vi "Regler FT-IR.vi"(7 "Index":i32, 8 "Fehler":errorcluster caption="Fehler (Eingang)") -> (0 "Fehler (Ausgang)":errorcluster)   [LabVIEW 2020, in "Regler.lvlib" / "Druckregler.lvlib"]
uses:
  Druckregler.lvlib
  Verwaltung/Verwaltung - cRIO.lvlib
  Aktionen Param. Druckregler.ctl
  Visualisierungs Elemente/Zahlen-Eingabefeld.ctl
  Allgemein/Allgemein.lvlib
  Allgemein/Aktionen FGV Dichtheitstest.ctl
  Aktionen Interne Werte.ctl
  Konfig-Dateien/Konfig-Dateien.lvlib
  Verwaltung/FGV IN Aktionen.ctl
  Konfig-Dateien/FGV Betriebsdaten Aktionen.ctl
  Verwaltung/FGV OUT Aktionen.ctl
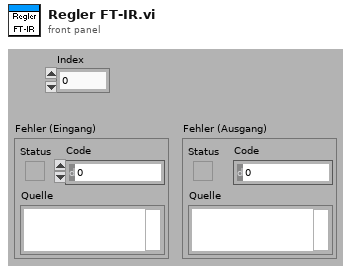
[diagram p1: front panel]
types:
  T1 = typedef "Verwaltung - cRIO.lvlib/FGV OUT Aktionen.ctl" = enum16{"lesen", "ANA OUT", "DO 0-31", "DO 32-47"}
  T2 = typedef "Konfig-Dateien.lvlib/FGV Betriebsdaten Aktionen.ctl" = enum16{"lesen", "Anlagengrenzw.", "PID Param.", "Sonstige", "Sensor Para."}
  T3 = typedef "Verwaltung - cRIO.lvlib/FGV IN Aktionen.ctl" = enum16{"lesen", "DI", "AI", "Fühler Br.", "TC", "Fühler Br. TC"}
  T4 = typedef "Regler.lvlib/Druckregler.lvlib/Aktionen Interne Werte.ctl" = enum16{"lesen", "FT-IR", "Ausgang", "Pumpe", "laden", "speichern", "Änderung?", "Druck Kalter Block", "Dichtheitstest"}
  T5 = typedef "Allgemein.lvlib/Aktionen FGV Dichtheitstest.ctl" = enum16{"lesen", "schreiben"}
  T6 = typedef "Zahlen-Eingabefeld.ctl" = sgl
  T7 = typedef "Regler.lvlib/Druckregler.lvlib/Aktionen Param. Druckregler.ctl" = enum16{"lesen", "schreiben", "Regler FT-IR", "Regler Ausgang", "Regler Durchfluss", "Regler PMA", "Regler NDIR", "Regler Filterblock", "Regler Gaskühler", "Regler Kalter Block"}
  T8 = typedef "Anlagengrenzwerte.lvlib/Anlagen-Grenzwerte Anzeige.ctl" = cluster{"Eingangsdruck FT-IR:":T9, "Durchfluss FT-IR:":T9, "Druck Ausgang:":T9, "Druck Kalter Block:":T9, "Heizleitungen intern:":T9, "Heizleitung zu FT-IR:":T9, "Heizung Filterblock:":T9, "Heizung Pumpe:":T9, "Heizleitung Extern SP1:":T9, "Heizleitung Extern SP2:":T9, "FT-IR Heizung Messzelle:":T9, "Schaltschranktemperatur:":T9, "Gaskühler:":T9, "Heizung VFE 2:":T9}
  T9 = typedef "Anlagengrenzwerte.lvlib/Anlagen-Parameter Anzeige.ctl" = cluster{"Sollwert":sgl, "Warn-Min":sgl, "Warn-Max":sgl, "Abschalt-Min":sgl, "Abschalt-Max":sgl, "Regler":u16}
  T10 = cluster{"AI0: Durchfluss FT-IR":sgl, "AI1: Druck Ausgang":sgl, "AI2: Umgebungsdruck":sgl, "AI3: Druck FT-IR":sgl, "AI4: Druck CalGas":sgl, "AI5: Reserve":sgl, "AI6: Reserve":sgl, "AI7: Reserve":sgl, "Rohwert Durchfluss FT-IR":sgl, "Rohwert Druck Ausgang":sgl, "Rohwert Umgebungsdruck":sgl, "Rohwert Druck FT-IR":sgl, "Schaltschrank":sgl, "Filter":sgl, "Pumpe":sgl, "HL BMP zu Filter":sgl, "HL zu FT-IR":sgl, "HL Extern SP1":sgl, "Reserve":sgl, "Reserve":sgl, "Reserve":sgl, "Reserve":sgl, "Reserve":sgl, "Reserve":sgl, "FT-IR":sgl, "Reserve":sgl, "Reserve":sgl, "Reserve":sgl}
  T11 = typedef "Verwaltung - cRIO.lvlib/Digital Ausgaenge 0-31.ctl" = cluster{"O0: Druckluft Versorgung":bool, "O1: (FB Eingang 1)":bool, "O2: Kühlung FT-IR EIN":bool, "O3: (FB Bypass)":bool, "O4: (FB CalGas)":bool, "O5: (FB spülen/UL)":bool, "O6: (FB zum FT-IR)":bool, "O7: (FB zum FID)":bool, "O8: (FB Reserve)":bool, "O9: (FB Reserve)":bool, "O10: (FB Umgebungsluft FID)":bool, "O11: (FB zum Gaskühler)":bool, "O12: FB Stickstoff zu FT-IR":bool, "O13: (FB Druckluft/UL)":bool, "O14: (Purifier deaktivieren)":bool, "O15: (Umschaltung Purifier/Stickstoff)":bool, "O16: N2 Einblasung":bool, "O17: LSP LN2 Nachfüllung":bool, "O18: (Reserve)":bool, "O19: (Pumpe Eingang1)":bool, "O20: (Pumpe Eingang2)":bool, "O21: (Pumpe Spülen1)":bool, "O22: (Pumpe Spülen2)":bool, "O23: (Reserve)":bool, "O24: CalGas 1":bool, "O25: CalGas 2":bool, "O26: CalGas 3":bool, "O27: Stickstoff aufschalten":bool, "O28: CG zu PNS":bool, "O29: FTIR Standby Spülung":bool, "O30: (Reserve)":bool, "O31: (Purifier regenerieren)":bool}
  T12 = cluster{"Numerisch":sgl, "Numerisch":sgl, "Numerisch":sgl, "Numerisch":sgl, "Numerisch":sgl}
  T13 = typedef "Regler.lvlib/Druckregler.lvlib/Regler Interne Werte.ctl" = cluster{"PV":sgl, "D-action":sgl, "Error":sgl, "I-action":sgl, "OUT":sgl}
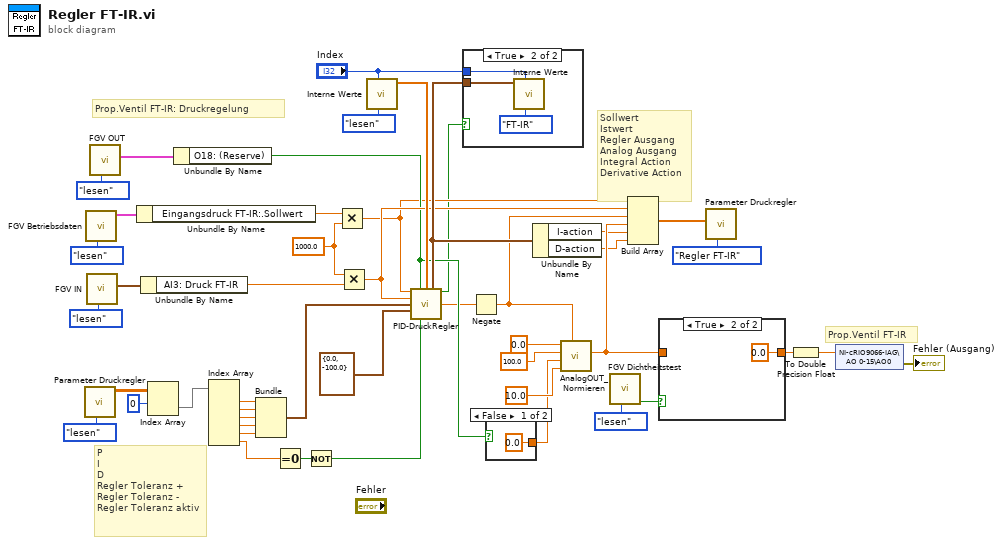
[diagram p0: block diagram]
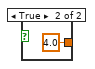
[diagram p4: hidden frame]
diagram:
  w25 = T6 1000.0 ("y")
  # "Prop.Ventil FT-IR"
  # "Prop.Ventil FT-IR: Druckregelung"
  # "Sollwert\nIstwert\nRegler Ausgang\nAnalog Ausgang\nIntegral Action\nDerivative Action"
  # "P\nI\nD\nRegler Toleranz +\nRegler Toleranz -\nRegler Toleranz aktiv"
  n1 = call "Parameter Druckregler.vi"("Aktionen"=Aktionen_Param._Druckregler."lesen") -> ("Regleparameter"=w30:sgl[][])  [unwired: 7 in, 3 out]
  n2 = call "FGV Betriebsdaten.vi"("Aktionen"=FGV_Betriebsdaten_Aktionen."lesen") -> ("Anlagen-Grenzwerte"=w2:T8)  [unwired: 7 in, 3 out]
  n3 = call "FGV IN.vi"("Aktion"=FGV_IN_Aktionen."lesen") -> ("Analog Eingänge"=w1:T10)  [unwired: 8 in, 2 out]
  n4 = call "FGV OUT.vi"("Aktion"=FGV_OUT_Aktionen."lesen") -> ("DO 0-31"=w3:T11)  [unwired: 7 in, 3 out]
  n5 = Unbundle By Name(w2) -> ("Eingangsdruck FT-IR:.Sollwert"=w26:sgl)
  n6 = Unbundle By Name(w1) -> ("AI3: Druck FT-IR"=w24:sgl)
  n7 = Index Array(array=w30, index (row)=0 ("Deaktivierter Index (Spalte)")) -> (element=w29:sgl[])  [unwired: 1 in]
  n8 = Unbundle By Name(w3) -> ("O18: (Reserve)"=w16:bool)
  n9 = Index Array(array=w29) -> (element #1=w41:sgl, element #2=w40:sgl, element #3=w39:sgl, element #4=w38:sgl, element #5=w37:sgl, element #6=w13:sgl)  [unwired: 6 in]
  n10 = Bundle("Numerisch"=w41, "Numerisch"=w40, "Numerisch"=w39, "Numerisch"=w38, "Numerisch"=w37) -> (w35:T12)  [unwired: 1 in]
  n11 = Equal To 0?(x=w13) -> (x = 0?=w36:bool)
  n12 = Not(x=w36) -> (.not. x?=w34:bool)
  n13 = Multiply(x=w26, y=w25) -> (x*y=w15:T6)
  n14 = Multiply(x=w25, y=w24) -> (x*y=w23:T6)
  n15 = call "Interne Werte.vi"("Aktionen Interne Werte"=Aktionen_Interne_Werte."lesen", "Index"="Index") -> ("FT-IR"=w47:sgl[])  [unwired: 4 in, 5 out]
  n16 = call "PID-DruckRegler.vi"("Sollwert"=w15, "Regler EIN"=w16, "Regler Interne Werte"=w47, "Istwert"=w23, "PID-Parameter"=w35, "output range"=cluster{"output high":dbl, "output low":dbl} {"output high"=0.0, "output low"=-100.0}, "Regler Toleranz verwenden?"=w34) -> ("Regler Interne Werte"=w46:T13, "Interne Werte speichern"=w10:bool, "Output"=w14:sgl)  [unwired: 6 in]
  n17 = case shown="True" w10 {
    tunnel: "Index" -> [_ w49]
    tunnel: w46 -> [_ w48]
    frame False {
    }
    frame True {
      n18 = call "Interne Werte.vi"("Aktionen Interne Werte"=Aktionen_Interne_Werte."FT-IR", "Index"=w49, "Regler Interne Werte"=w48) -> ()  [unwired: 3 in, 6 out]
    }
  }
  n19 = Negate(x=w14) -> (-x=w17:sgl)
  n20 = case shown="False" w16 {
    tunnel: [sgl 0.0 ("Untergrenze") sgl 4.0 ("Untergrenze")] -> w33
    frame False {
    }
    frame True {
    }
  }
  n21 = Unbundle By Name(w46) -> ("I-action"=w9:sgl, "D-action"=w8:sgl)
  n22 = call "AnalogOUT_Normieren.vi"("Analogwert"=w17, "Obergrenze"=sgl 10.0, "Untergrenze"=w33, "Max Analogwert"=sgl 100.0, "Min Analogwert"=sgl 0.0) -> ("Normierter Wert"=w20:sgl)  [unwired: 6 in]
  n23 = call "FGV Dichtheitstest.vi"("Aktionen"=Aktionen_FGV_Dichtheitstest."lesen") -> ("Dichtheitstest?"=w18:bool)  [unwired: 9 in, 1 out]
  n24 = Build Array(w15, w23, w17, w20, w9, w8) -> (w28:T6[])
  n25 = case shown="True" w18 {
    tunnel: w20 -> [w53 _]
    tunnel: [w53 sgl 0.0 ("Normierter Wert")] -> w19
    frame False {
    }
    frame True {
    }
  }
  n26 = call "Parameter Druckregler.vi"("Aktionen"=Aktionen_Param._Druckregler."Regler FT-IR", "Werte FT-IR"=w28) -> ()  [unwired: 6 in, 4 out]
  n27 = To Double Precision Float(number=w19) -> (double precision float=w22:dbl)
  n28 = shared-variable "NI-cRIO9066-IAG\\AO 0-15\\AO0"(w22) -> (error out=→"Fehler (Ausgang)":errorcluster)  [unwired: 1 in]
